vi "Find Objects.vi"(8 "Error In":errorcluster, 9 "Game Ball":T2(plugin-control), 10 "Blue Team":T2(plugin-control), 11 "Red Team":T2(plugin-control)) -> (0 "Error Out":errorcluster, 1 "Ball Object":T1, 2 "Blue Objects":T1, 3 "Red Objects":T1)   [LabVIEW 2018]
uses:
  Image Object.ctl
  <vilib>/vision/Image Controls.llb/IMAQ Image.ctl
  <vilib>/vision/NI_Vision_Development_Module.lvlib
panel:
  out "Game Ball (Searched)":T2(plugin-control)
  out "Red Team (Searched)":T2(plugin-control)
  out "Blue Team (Searched)":T2(plugin-control)
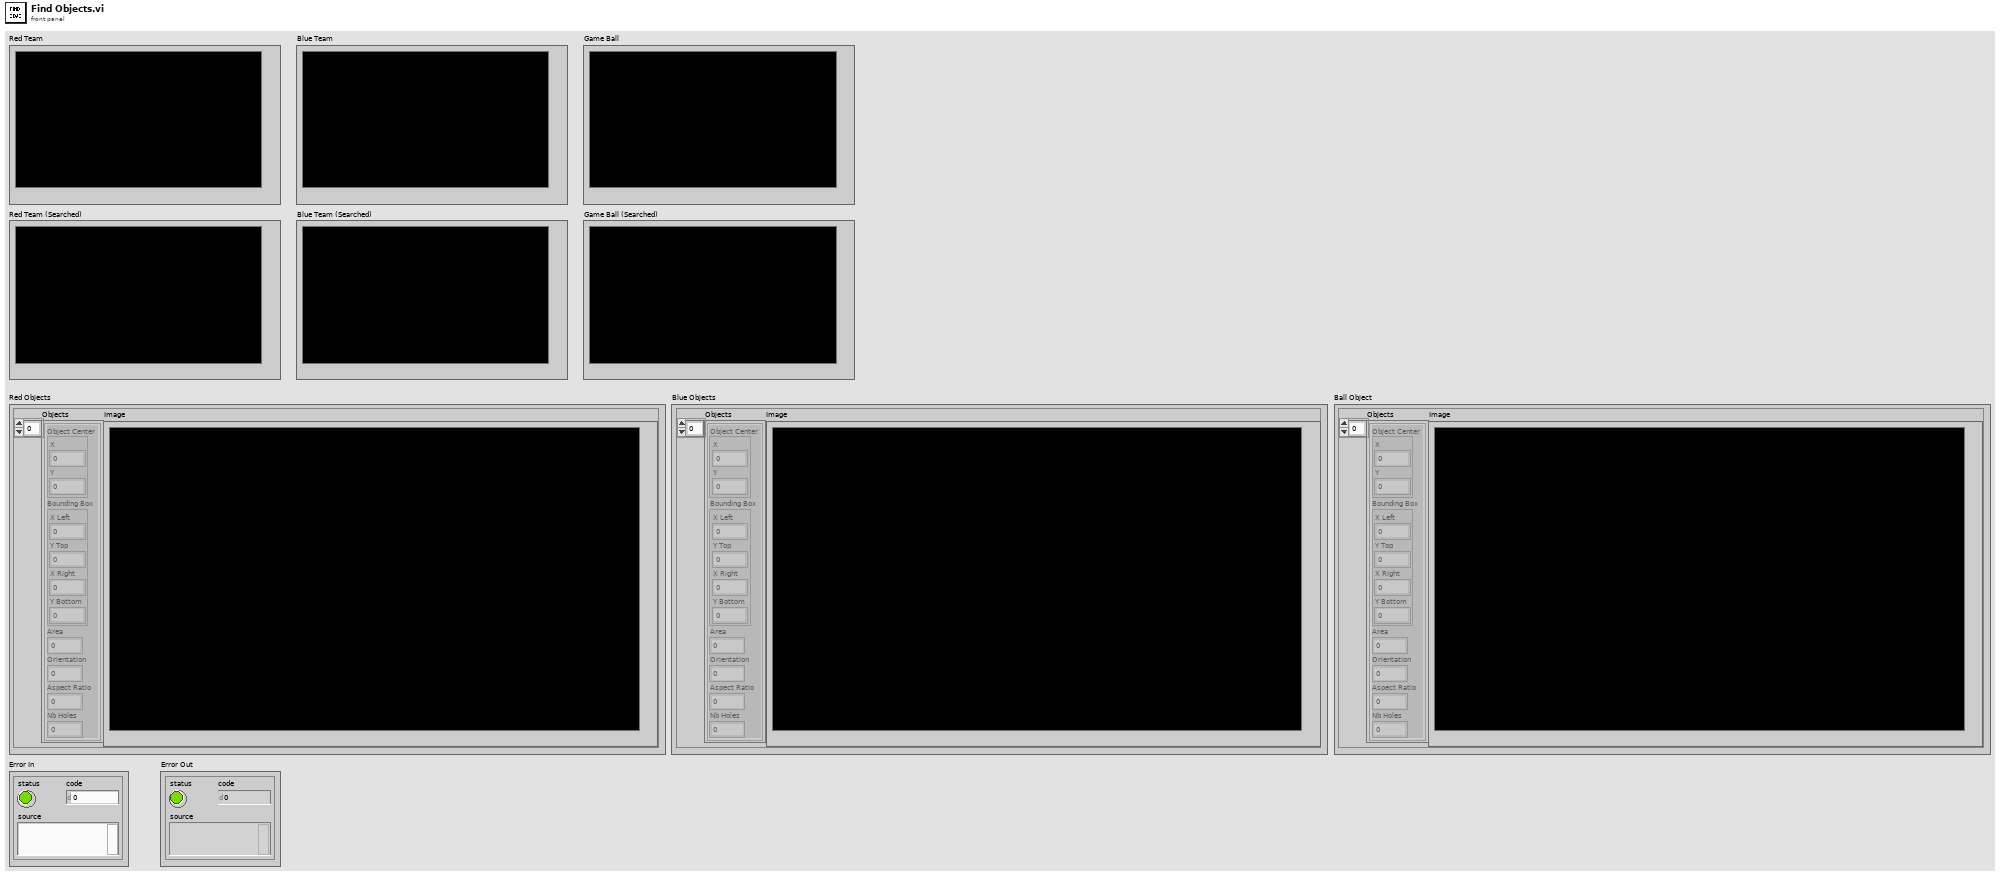
[diagram p1: front panel]
types:
  T1 = typedef "Image Object.ctl" = cluster{"Objects":cluster{"Object Center":cluster{"X":sgl, "Y":sgl}, "Bounding Box":cluster{"X Left":i32, "Y Top":i32, "X Right":i32, "Y Bottom":i32}, "Area":sgl, "Orientation":sgl, "Aspect Ratio":sgl, "Nb Holes":i32}[], "Image":T2}
  T2 = typedef "IMAQ Image.ctl" = refnum<image>
  T3 = cluster{"Objects":u16, "Threshold":i32, "Reject Border":bool, "Fill Holes":bool, "Min Object Size":bool, "Min Size":i32, "Max Object Size":bool, "Max Size":i32, "Show Search Area":bool, "Show Center":bool, "Show Bounding Box":bool}
  T4 = enum32{"AutoM", "Close", "Dilate", "Erode", "Gradient", "Gradient in", "Gradient out", "HitMiss", "Open", "PClose", "POpen", "Thick", "Thin"}
  T5 = cluster{"Object Center":cluster{"X":sgl, "Y":sgl}, "Bounding Box":cluster{"X Left":i32, "Y Top":i32, "X Right":i32, "Y Bottom":i32}, "Area":sgl, "Orientation":sgl, "Aspect Ratio":sgl, "Nb Holes":i32}[]
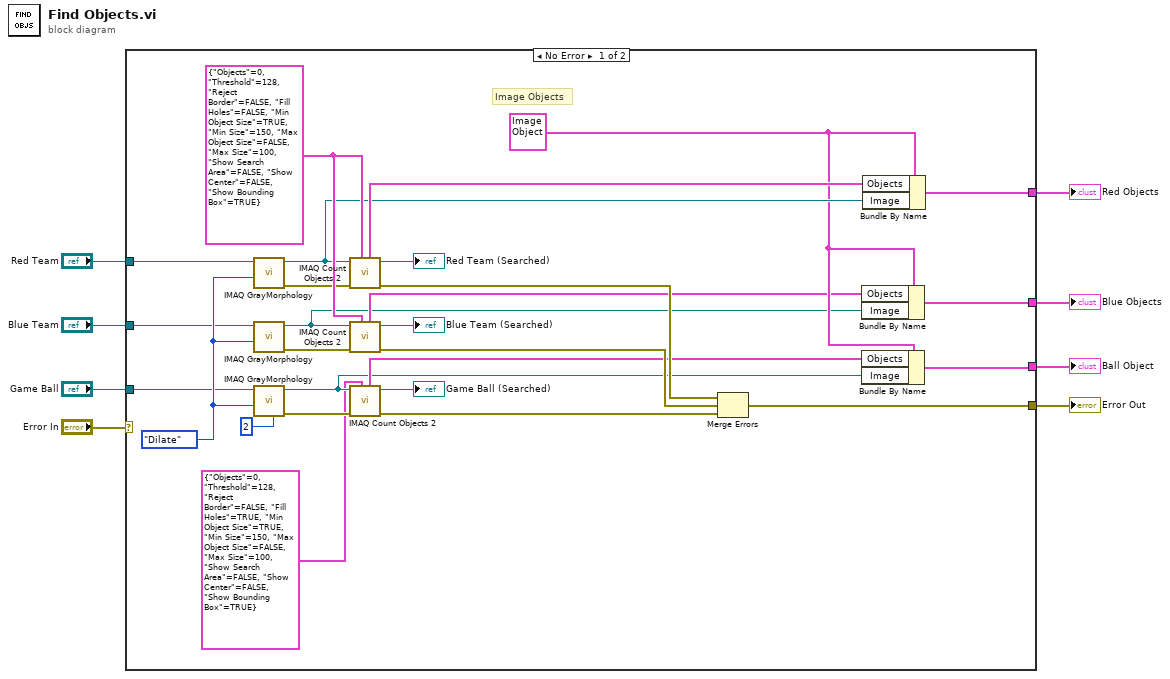
[diagram p0: block diagram]
diagram:
  n1 = case shown="No Error" "Error In" {
    selector: "Error In" -> [_ w36]
    tunnel: "Red Team" -> [w29 _]
    tunnel: "Blue Team" -> [w23 _]
    tunnel: "Game Ball" -> [w24 _]
    tunnel: [w30 w36] -> w4
    tunnel: [w14 _] -> w3
    tunnel: [w13 _] -> w2
    tunnel: [w12 _] -> w1
    frame No Error {
      w18 = T1 {"Objects"=[], "Image"=refnum} ("Red Objects 2")
      w25 = T4."Dilate" ("Operation")
      w34 = T3 {"Objects"=0, "Threshold"=128, "Reject Border"=FALSE, "Fill Holes"=FALSE, "Min Object Size"=TRUE, "Min Size"=150, "Max Object Size"=FALSE, "Max Size"=100, "Show Search Area"=FALSE, "Show Center"=FALSE, "Show Bounding Box"=TRUE} ("Settings")
      # "Image Objects"
      n2 = call "IMAQ GrayMorphology"("Operation"=w25, "Image Src"=w29) -> ("error out"=w28:errorcluster, "Image Dst Out"=w19:T2)  [unwired: 8 in]
      n3 = call "IMAQ GrayMorphology"("Operation"=w25, "Image Src"=w23) -> ("error out"=w27:errorcluster, "Image Dst Out"=w11:T2)  [unwired: 8 in]
      n4 = call "IMAQ GrayMorphology"("Number of iterations (1)"=2, "Operation"=w25, "Image Src"=w24) -> ("error out"=w26:errorcluster, "Image Dst Out"=w15:T2)  [unwired: 7 in]
      n5 = call "IMAQ Count Objects 2"("Settings"=w34, "error in (no error)"=w28, "Image"=w19) -> ("error out"=w33:errorcluster, "Image Out"=→"Red Team (Searched)":T2, "Objects"=w20:T5)  [unwired: 4 in, 2 out]
      n6 = call "IMAQ Count Objects 2"("Settings"=w34, "error in (no error)"=w27, "Image"=w11) -> ("error out"=w32:errorcluster, "Image Out"=→"Blue Team (Searched)":T2, "Objects"=w17:T5)  [unwired: 4 in, 2 out]
      n7 = call "IMAQ Count Objects 2"("Settings"=T3 {"Objects"=0, "Threshold"=128, "Reject Border"=FALSE, "Fill Holes"=TRUE, "Min Object Size"=TRUE, "Min Size"=150, "Max Object Size"=FALSE, "Max Size"=100, "Show Search Area"=FALSE, "Show Center"=FALSE, "Show Bounding Box"=TRUE}, "error in (no error)"=w26, "Image"=w15) -> ("error out"=w31:errorcluster, "Image Out"=→"Game Ball (Searched)":T2, "Objects"=w16:T5)  [unwired: 4 in, 2 out]
      n8 = Merge Errors(w33, w32, w31) -> (w30:errorcluster)
      n9 = Bundle By Name(cluster=w18, "Objects"=w17, "Image"=w11) -> (w13:T1)
      n10 = Bundle By Name(cluster=w18, "Objects"=w16, "Image"=w15) -> (w12:T1)
      n11 = Bundle By Name(cluster=w18, "Objects"=w20, "Image"=w19) -> (w14:T1)
    }
    frame Error {
    }
  }
  "Error Out" <- w4
  "Red Objects" <- w3
  "Blue Objects" <- w2
  "Ball Object" <- w1
